vi "Get Therm Calibration File.vi"(0 "Calibration (Empty gives dialog)":string) -> (1 "Calbration Name":string, 2 "Temperature":dbl[](array[numeric]) format="%.3f", 3 "Resistance":dbl[](array[numeric]) format="%.2f", 4 "error out":errorcluster)   [LabVIEW 2020]
doc: "This VI reads a calibration file (or asks for one at a prompt) and reads the temperatures and resistances from it. The file may have comments which are lines starting with the # character. The data is returned sorted in increasing Resistance values. The first line of the file is returned as the calibration name.\nScott Hannahs, <sth@magnet.fsu.edu> NHMFL-FSU, May 2003"
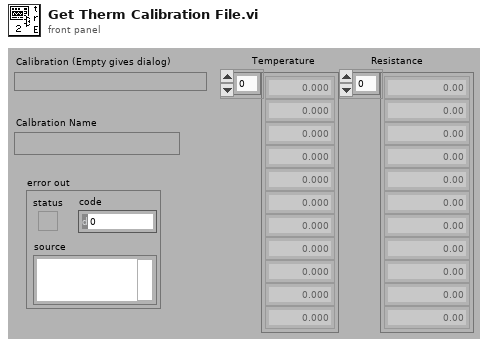
[diagram p1: front panel]
types:
  T1 = enum16{"read/write", "read-only", "write-only", "write-only (truncate)"}
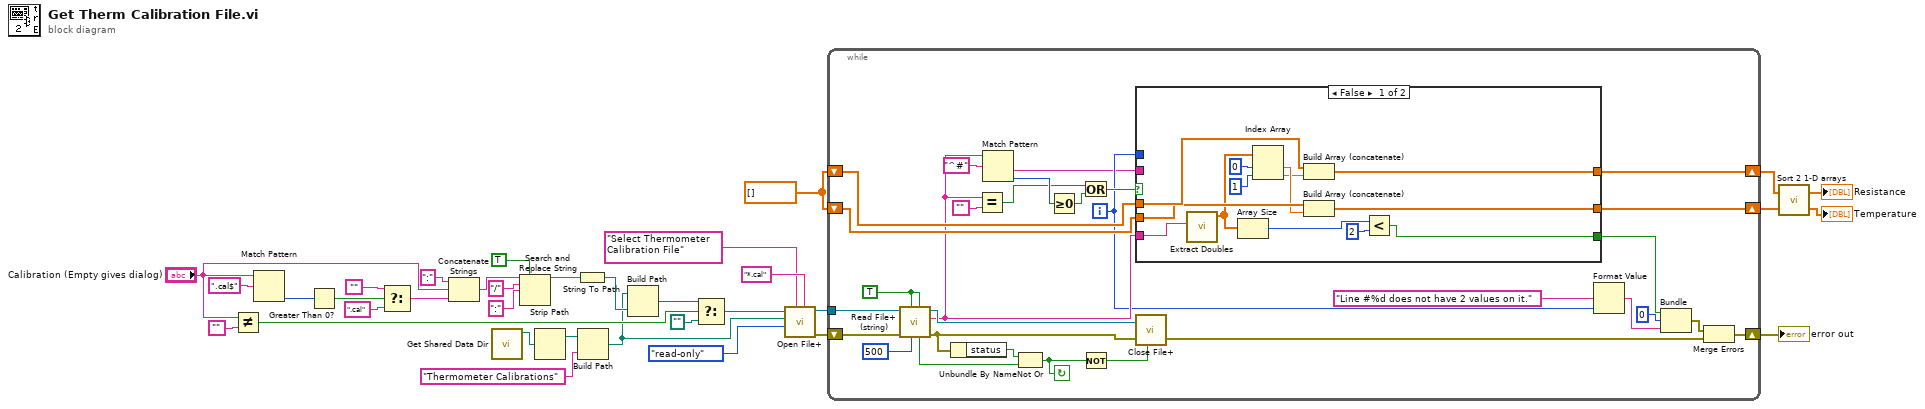
[diagram p0: block diagram]
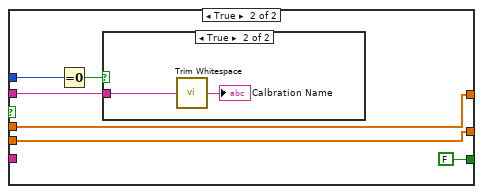
[diagram p2: hidden frame]
diagram:
  w1 = dbl[] [] ("initialized array")
  n1 = Not Equal?(x="Calibration (Empty gives dialog)", y="") -> (x != y?=w10:bool)
  n2 = Match Pattern(string="Calibration (Empty gives dialog)", regular expression=".cal$") -> (offset past match=w28:i32)  [unwired: 1 in, 3 out]
  n3 = Greater Than 0?(x=w28) -> (x > 0?=w7:bool)
  n4 = Select(t="", s=w7, f=".cal") -> (s? t:f=w8:string)
  n5 = Concatenate Strings(":" ("string"), "Calibration (Empty gives dialog)", w8) -> (w17:string)
  n6 = call "Get Shared Data Dir.vi"() -> ("Data Directory Path"=w21:path)  [unwired: 2 in, 1 out]
  n7 = Search and Replace String(replace all?=TRUE ("replace all? (F)"), input string=w17, search string="/", replace string=":" ("replace string (\"\")")) -> (result string=w18:string)  [unwired: 4 in, 3 out]
  n8 = Strip Path(path=w21) -> (stripped path=w9:path)  [unwired: 1 out]
  n9 = String To Path(string=w18) -> (path=w20:path)
  n10 = Build Path(base path=w9, name or relative path="Thermometer Calibrations") -> (appended path=w3:path)
  n11 = Build Path(base path=w3, name or relative path=w20) -> (appended path=w4:path)
  n12 = Select(t=w4, s=w10, f=path "") -> (s? t:f=w12:path)
  n13 = call <vilib>:"Open File+.vi"("[pattern]"="*.cal", "prompt"="Select Thermometer Calibration File", "open mode (read-only:1)"=T1."read-only", "start path (Not A Path)"=w3, "file path (\" \")"=w12) -> ("error out"=w31:errorcluster, "refnum"=w32:refnum<file>)  [unwired: 3 in, 2 out]
  n14 = while {
    shift-left: w1 -> [w58]
    shift-right: [w55] -> w24
    shift-left: w1 -> [w57]
    shift-right: [w56] -> w25
    shift-left: w31 -> [w63]
    shift-right: [w47] -> w30
    tunnel: w32 -> [w64]
    i -> [w37]
    stop <- w50 continue-if-true
    w62 = TRUE
    n15 = call <vilib>:"Read File+ (string).vi"("convert eol? (no:F)"=w62, "count"=500, "line mode (characters:F)"=w62, "error in (no error)"=w63, "refnum"=w64) -> ("error out"=w52:errorcluster, "string"=w41:string, "dup refnum"=w49:refnum<file>, "EOF?"=w53:bool)  [unwired: 2 in, 1 out]
    n16 = Unbundle By Name(w52) -> ("status"=w54:bool)
    n17 = Equal?(x=w41, y="") -> (x = y?=w42:bool)
    n18 = Match Pattern(string=w41, regular expression="^#") -> (after substring=w35:string, offset past match=w60:i32)  [unwired: 1 in, 2 out]
    n19 = Not Or(1:w53, 2:w54) -> (0:w50:bool)
    n20 = Greater Or Equal To 0?(x=w60) -> (x >= 0?=w59:bool)
    n21 = Or(x=w42, y=w59) -> (x .or. y?=w43:bool)
    n22 = Not(x=w50) -> (.not. x?=w51:bool)
    n23 = case shown="False" w43 {
      tunnel: [w73 w83] -> w55
      tunnel: w58 -> [w76 w83]
      tunnel: [w72 w82] -> w56
      tunnel: w57 -> [w75 w82]
      tunnel: w41 -> [w77 _]
      tunnel: [w67 FALSE] -> w45
      tunnel: w35 -> [_ w80]
      tunnel: w37 -> [_ w79]
      frame False {
        n24 = call "Extract Doubles.vi"("String"=w77) -> ("Data"=w70:dbl[])  [unwired: 5 in, 1 out]
        n25 = Array Size(array=w70) -> (size(s)=w69:i32)
        n26 = Index Array(array=w70, index #1=0, index #2=1) -> (element #1=w74:dbl, element #2=w65:dbl)
        n27 = Build Array (concatenate)(w76, w65) -> (w73:dbl[])
        n28 = Build Array (concatenate)(w75, w74) -> (w72:dbl[])
        n29 = Less?(x=w69, y=2) -> (x < y?=w67:bool)
      }
      frame True {
        n30 = Equal To 0?(x=w79) -> (x = 0?=w78:bool)
        n31 = case shown="True" w78 {
          tunnel: w80 -> [_ w85]
          frame False {
          }
          frame True {
            n32 = call <vilib>:"Trim Whitespace.vi"("string"=w85) -> ("trimmed string"=→"Calbration Name":string)  [unwired: 1 in]
          }
        }
      }
    }
    n33 = call <vilib>:"Close File+.vi"("error in (no error)"=w52, "close when? (now:T)"=w51, "refnum"=w49) -> ("error out"=w48:errorcluster)  [unwired: 2 in, 2 out]
    n34 = Format Value(format string="Line #%d does not have 2 values on it.", value (0)=w37) -> (output string=w39:string)  [unwired: 1 in]
    n35 = Bundle(w45, 0, "output string"=w39) -> (w46:cluster{bool, i32, "output string":string})  [unwired: 1 in]
    n36 = Merge Errors(w46, w48) -> (w47:errorcluster)
  }
  "error out" <- w30
  n37 = call "Sort 2 1-D arrays.vi"("Array 2"=w25, "Array 1"=w24) -> ("Array 2"=→"Temperature":dbl[], "Array 1"=→"Resistance":dbl[])
